vi "executeScript.vi"(0 "script":string[][](array[string]), 2 "lastUpdate":u32, 3 "error in (no error)":errorcluster) -> (7 "scriptOut":string[][](array[string]), 9 "lastUpdate 2":u32, 10 "error out":errorcluster)   [LabVIEW 2018]
uses:
  Strict Type Controls/Command.ctl
  classes/Variable Manager/VariableManager_Bool.vi
  classes/Variable Manager/VariableManager_Double.vi
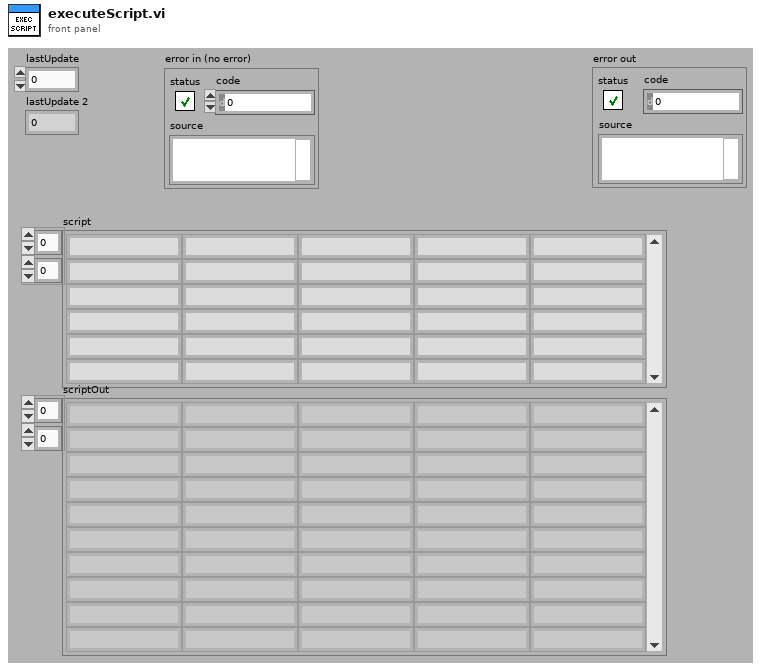
[diagram p1: front panel]
types:
  T1 = typedef "Command.ctl" = enum16{"selectChannel", "setDCVoltage", "setDCCurrent", "setVoltageSteps", "wait", "setWavelength", "setWavelengthSteps"}
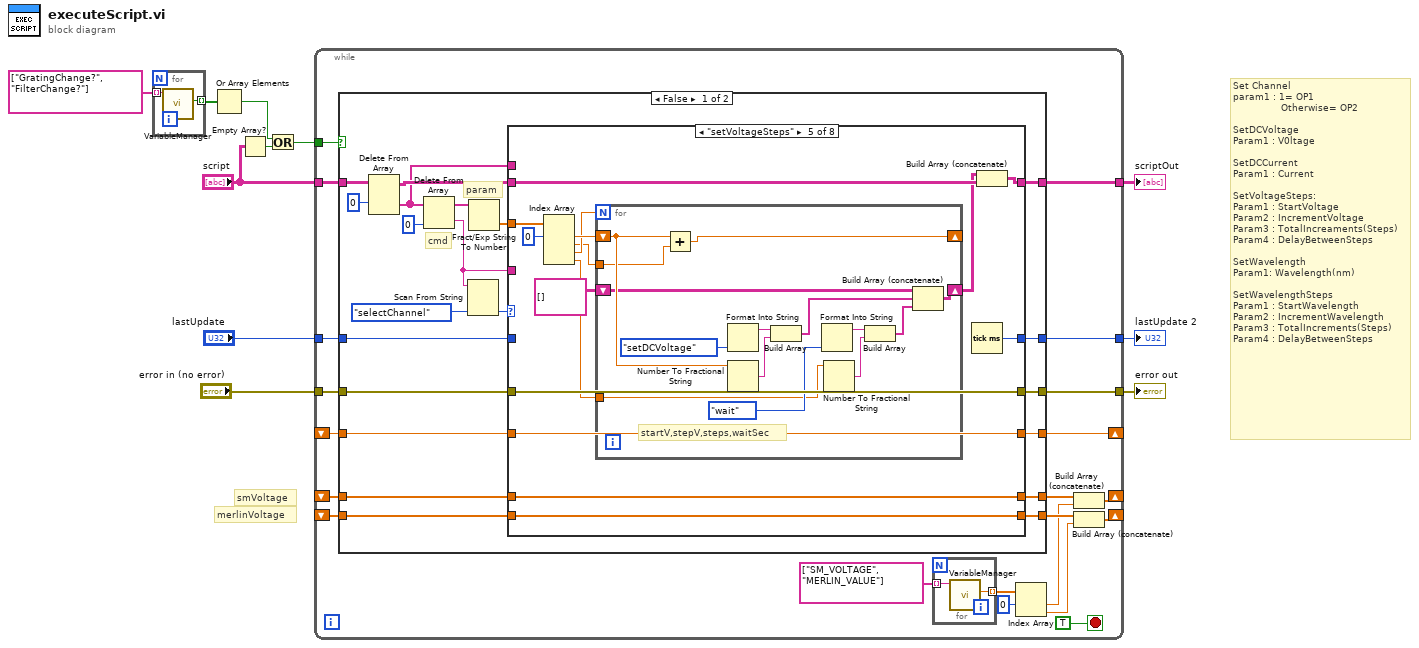
[diagram p0: block diagram]
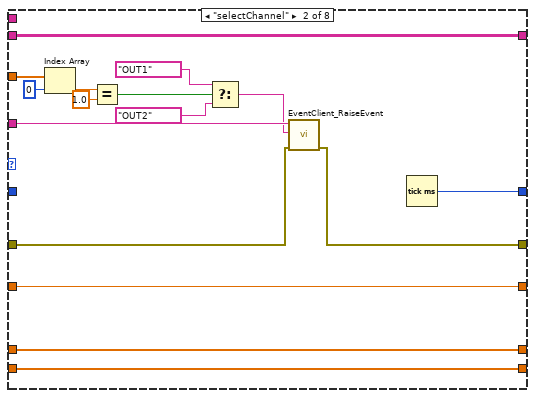
[diagram p3: hidden frame]
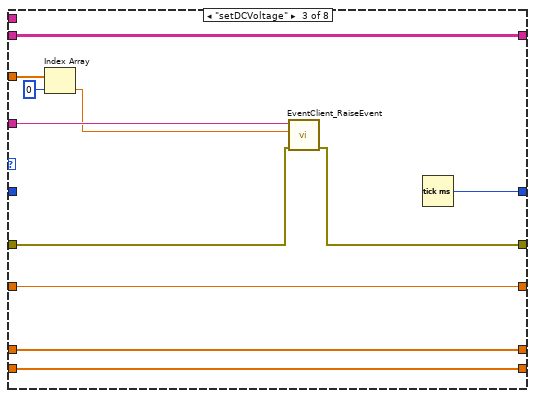
[diagram p4: hidden frame]
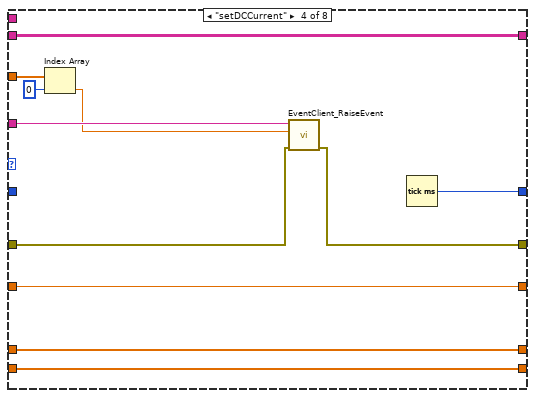
[diagram p5: hidden frame]
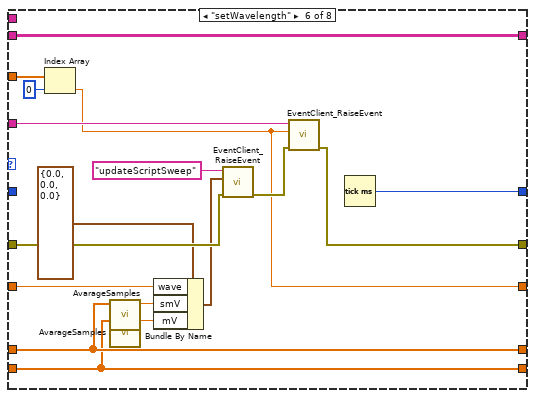
[diagram p6: hidden frame]
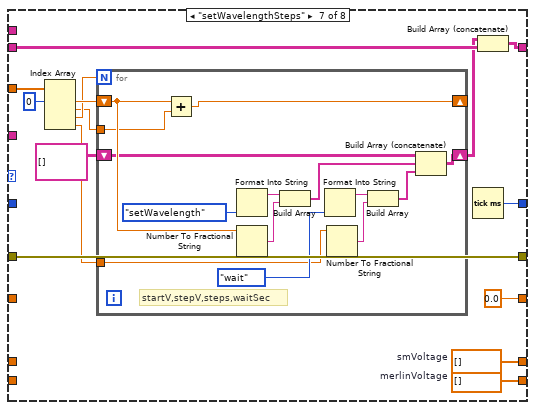
[diagram p7: hidden frame]
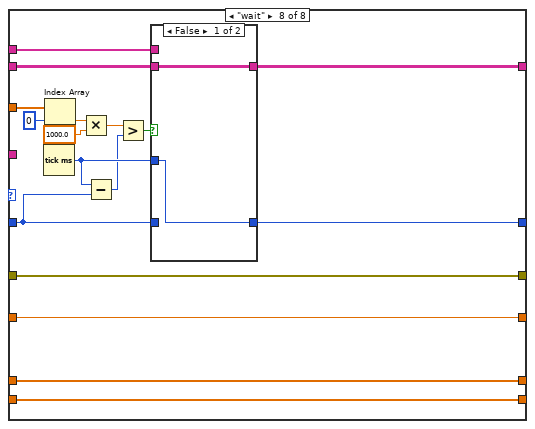
[diagram p8: hidden frame]
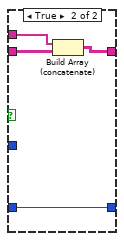
[diagram p9: hidden frame]
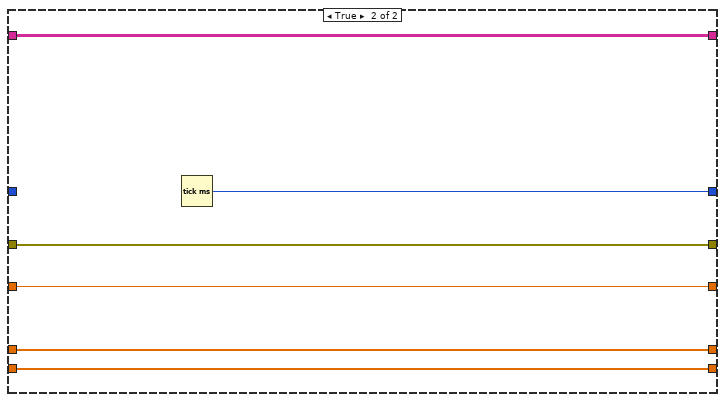
[diagram p10: hidden frame]
diagram:
  # "Set Channel\nparam1 : 1= OP1\n                Otherwise= OP2\n\nSetDCVoltage\nParam1 : V0ltage\n\nSetDCCurrent\nParam1 : Current\n\nSetVoltageSteps:\nParam1 : StartVoltage\nParam2 : IncrementVoltage\nParam3 : TotalIncreaments(Steps)\nParam4 : DelayBetweenSteps\n\nSetWavelength\nParam1: Wavelength(nm)\n\nSetWavelengthSteps\nParam1 : StartWavelength\nParam2 : IncrementWavelength\nParam3 : TotalIncrements(Steps)\nParam4 : DelayBetweenSteps"
  # "merlinVoltage"
  # "smVoltage"
  n1 = for {
    tunnel: string[] ["GratingChange?", "FilterChange?"] -> [w13] mode=indexing
    tunnel: [w12] -> w3 mode=indexing
    n2 = call-poly "VariableManager.vi"("Tag"=w13) -> ("Value out"=w12:bool)  [unwired: 7 in, 3 out]
  }
  n3 = Or Array Elements(Boolean array=w3) -> (logical OR=w1:bool)
  n4 = Empty Array?(array="script") -> (empty?=w8:bool)
  n5 = Or(x=w1, y=w8) -> (x .or. y?=w4:bool)
  n6 = while {
    tunnel: "script" -> [w34]
    tunnel: [w33] -> w10
    tunnel: "error in (no error)" -> [w32]
    tunnel: [w31] -> w7
    tunnel: "lastUpdate" -> [w30]
    tunnel: [w29] -> w5
    tunnel: w4 -> [w28]
    shift-right: [w20] -> _
    shift-left: _ -> [w26]
    shift-right: [w19] -> _
    shift-left: _ -> [w25]
    shift-right: [w21] -> _
    shift-left: _ -> [w22]
    stop <- TRUE stop-if-true
    n7 = case shown="False" w28 {
      tunnel: w34 -> [w57 w205]
      tunnel: [w47 w205] -> w31
      tunnel: [w52 w204] -> w33
      tunnel: w32 -> [w53 w204]
      tunnel: w30 -> [w45 _]
      tunnel: [w43 w203] -> w29
      tunnel: w26 -> [w42 w201]
      tunnel: w25 -> [w41 w200]
      tunnel: [w40 w201] -> w24
      tunnel: [w39 w200] -> w23
      tunnel: w22 -> [w38 w202]
      tunnel: [w37 w202] -> w21
      frame False {
        # "cmd"
        # "param"
        n8 = Delete From Array(array=w57, index (row)=0) -> (deleted portion=w44:string[], array with subset deleted=w48:string[][])  [unwired: 2 in]
        n9 = Delete From Array(array=w44, index=0) -> (deleted portion=w49:string, array with subset deleted=w51:string[])  [unwired: 1 in]
        n10 = Scan From String(input string=w49, default 1=Command."selectChannel" ("Command")) -> (output 1=w54:T1)  [unwired: 3 in, 3 out]
        n11 = Fract/Exp String To Number(string=w51) -> (number=w50:dbl[])  [unwired: 3 in, 1 out]
        n12 = case shown="\"setVoltageSteps\"" w54 {
          tunnel: w53 -> [w61 w70 w87 w98 w115 w140 w161 w190]
          tunnel: [w61 w69 w86 w97 w115 w144 w161 w190] -> w52
          tunnel: w50 -> [_ w79 w90 w101 w110 w147 w156 w193]
          tunnel: w49 -> [_ w74 w88 w99 _ w145 _ _]
          tunnel: w48 -> [w63 w68 w84 w95 w109 w143 w155 w191]
          tunnel: [w63 w68 w84 w95 w108 w143 w154 w187] -> w47
          tunnel: w45 -> [w62 _ _ _ _ _ _ w183]
          tunnel: w44 -> [_ _ _ _ _ _ _ w186]
          tunnel: [w62 w67 w83 w94 w105 w142 w151 w184] -> w43
          tunnel: w42 -> [w59 w65 w81 w92 w104 w134 _ w178]
          tunnel: w41 -> [w58 w64 w80 w91 w102 w133 _ w177]
          tunnel: [w59 w65 w81 w92 w104 w134 w150 w178] -> w40
          tunnel: [w58 w64 w80 w91 w102 w133 w149 w177] -> w39
          tunnel: w38 -> [w60 w66 w82 w93 w103 w137 _ w179]
          tunnel: [w60 w66 w82 w93 w103 w131 0.0 w179] -> w37
          frame Default {
          }
          frame "selectChannel" {
            n13 = Index Array(array=w79, index=0) -> (element=w77:dbl)
            n14 = Equal?(x=w77, y=1.0) -> (x = y?=w75:bool)
            n15 = Select(t="OUT1" ("Instrument Select (Output 1)"), s=w75, f="OUT2" ("Instrument Select (Output 1)")) -> (s? t:f=w71:string)
            n16 = call "EventClient_RaiseEvent.vi"("error in (no error)"=w70, "Data"=w71, "Event"=w74) -> ("error out"=w69:errorcluster)  [unwired: 8 in]
            n17 = Tick Count (ms)() -> (millisecond timer value=w67:u32)
          }
          frame "setDCVoltage" {
            n18 = Index Array(array=w90, index=0) -> (element=w85:dbl)
            n19 = call "EventClient_RaiseEvent.vi"("error in (no error)"=w87, "Data"=w85, "Event"=w88) -> ("error out"=w86:errorcluster)  [unwired: 8 in]
            n20 = Tick Count (ms)() -> (millisecond timer value=w83:u32)
          }
          frame "setDCCurrent" {
            n21 = Index Array(array=w101, index=0) -> (element=w96:dbl)
            n22 = call "EventClient_RaiseEvent.vi"("error in (no error)"=w98, "Data"=w96, "Event"=w99) -> ("error out"=w97:errorcluster)  [unwired: 8 in]
            n23 = Tick Count (ms)() -> (millisecond timer value=w94:u32)
          }
          frame "setVoltageSteps" {
            n24 = Index Array(array=w110, index #1=0 ("index")) -> (element #1=w114:dbl, element #2=w112:dbl, element #3=w113:dbl, element #4=w111:dbl)  [unwired: 3 in]
            n25 = for {
              N: w113 -> [_]
              shift-right: [w124] -> _
              shift-left: w114 -> [w126]
              tunnel: w112 -> [w125]
              tunnel: w111 -> [w122]
              shift-right: [w119] -> w106
              shift-left: string[][] [] -> [w118]
              # "startV,stepV,steps,waitSec"
              n26 = Add(x=w126, y=w125) -> (x+y=w124:dbl)
              n27 = Format Into String(Command."setDCVoltage" ("Command")) -> (resulting string=w130:string)  [unwired: 3 in, 1 out]
              n28 = Number To Fractional String(number=w126) -> (F-format string=w127:string)  [unwired: 3 in]
              n29 = Build Array(w130, w127) -> (w120:string[])
              n30 = Format Into String(Command."wait" ("Command")) -> (resulting string=w129:string)  [unwired: 3 in, 1 out]
              n31 = Number To Fractional String(number=w122) -> (F-format string=w123:string)  [unwired: 3 in]
              n32 = Build Array(w129, w123) -> (w121:string[])
              n33 = Build Array (concatenate)(w118, w120, w121) -> (w119:string[][])
            }
            n34 = Tick Count (ms)() -> (millisecond timer value=w105:u32)
            n35 = Build Array (concatenate)(w106, w109) -> (w108:string[][])
          }
          frame "setWavelength" {
            n36 = Index Array(array=w147, index=0) -> (element=w131:dbl)
            n37 = call "AvarageSamples.vi"("samples"=w134) -> ("Avg"=w135:dbl)  [unwired: 10 in]
            n38 = call "AvarageSamples.vi"("samples"=w133) -> ("Avg"=w136:dbl)  [unwired: 10 in]
            n39 = Bundle By Name(cluster=cluster{"wave":dbl, "smV":dbl, "mV":dbl} {"wave"=0.0, "smV"=0.0, "mV"=0.0}, "wave"=w137, "smV"=w135, "mV"=w136) -> (w132:cluster{"wave":dbl, "smV":dbl, "mV":dbl})
            n40 = call "EventClient_RaiseEvent.vi"("error in (no error)"=w140, "Data"=w132, "Event"="updateScriptSweep") -> ("error out"=w139:errorcluster)  [unwired: 8 in]
            n41 = call "EventClient_RaiseEvent.vi"("error in (no error)"=w139, "Data"=w131, "Event"=w145) -> ("error out"=w144:errorcluster)  [unwired: 8 in]
            n42 = Tick Count (ms)() -> (millisecond timer value=w142:u32)
          }
          frame "setWavelengthSteps" {
            w149 = dbl[] []  # merlinVoltage
            w150 = dbl[] []  # smVoltage
            n43 = Index Array(array=w156, index #1=0 ("index")) -> (element #1=w160:dbl, element #2=w158:dbl, element #3=w159:dbl, element #4=w157:dbl)  [unwired: 3 in]
            n44 = for {
              N: w159 -> [_]
              shift-right: [w170] -> _
              shift-left: w160 -> [w172]
              tunnel: w158 -> [w171]
              tunnel: w157 -> [w168]
              shift-right: [w165] -> w152
              shift-left: string[][] [] -> [w164]
              # "startV,stepV,steps,waitSec"
              n45 = Add(x=w172, y=w171) -> (x+y=w170:dbl)
              n46 = Format Into String(Command."setWavelength" ("Command")) -> (resulting string=w176:string)  [unwired: 3 in, 1 out]
              n47 = Number To Fractional String(number=w172) -> (F-format string=w173:string)  [unwired: 3 in]
              n48 = Build Array(w176, w173) -> (w166:string[])
              n49 = Format Into String(Command."wait" ("Command")) -> (resulting string=w175:string)  [unwired: 3 in, 1 out]
              n50 = Number To Fractional String(number=w168) -> (F-format string=w169:string)  [unwired: 3 in]
              n51 = Build Array(w175, w169) -> (w167:string[])
              n52 = Build Array (concatenate)(w164, w166, w167) -> (w165:string[][])
            }
            n53 = Tick Count (ms)() -> (millisecond timer value=w151:u32)
            n54 = Build Array (concatenate)(w152, w155) -> (w154:string[][])
          }
          frame "wait" {
            n55 = Tick Count (ms)() -> (millisecond timer value=w182:u32)
            n56 = Index Array(array=w193, index=0) -> (element=w189:dbl)
            n57 = Multiply(x=w189, y=1000.0) -> (x*y=w181:dbl)
            n58 = Subtract(x=w182, y=w183) -> (x-y=w180:u32)
            n59 = Greater?(x=w181, y=w180) -> (0:w185:bool)
            n60 = case shown="False" w185 {
              tunnel: w191 -> [w195 w199]
              tunnel: [w195 w198] -> w187
              tunnel: w186 -> [_ w197]
              tunnel: [w194 w196] -> w184
              tunnel: w183 -> [_ w196]
              tunnel: w182 -> [w194 _]
              frame False {
              }
              frame True {
                n61 = Build Array (concatenate)(w197, w199) -> (w198:string[][])
              }
            }
          }
        }
      }
      frame True {
        n62 = Tick Count (ms)() -> (millisecond timer value=w203:u32)
      }
    }
    n63 = for {
      tunnel: string[] ["SM_VOLTAGE", "MERLIN_VALUE"] ("State Array Out") -> [w36] mode=indexing
      tunnel: [w35] -> w17 mode=indexing
      n64 = call-poly "VariableManager.vi"("Tag"=w36) -> ("Value out"=w35:dbl)  [unwired: 6 in, 4 out]
    }
    n65 = Index Array(array=w17, index #1=0 ("index")) -> (element #1=w15:dbl, element #2=w14:dbl)  [unwired: 1 in]
    n66 = Build Array (concatenate)(w24, w15) -> (w20:dbl[])
    n67 = Build Array (concatenate)(w23, w14) -> (w19:dbl[])
  }
  "scriptOut" <- w7
  "error out" <- w10
  "lastUpdate 2" <- w5
